vi "Reset Alarm.vi"(8 "error in (no error)":errorcluster, 11 "FujiMotor in":refnum<class "FujiMotor.lvclass">) -> (0 "error out":errorcluster, 3 "FujiMotor out":refnum<class "FujiMotor.lvclass">)   [LabVIEW 2014, in "ALPHA5 RS485.lvlib" / "FujiMotor.lvclass"]
uses:
  FujiMotor.lvclass
  FujiMotor.lvclass/FujiMotor.ctl
  ALPHA5 RS485.lvlib
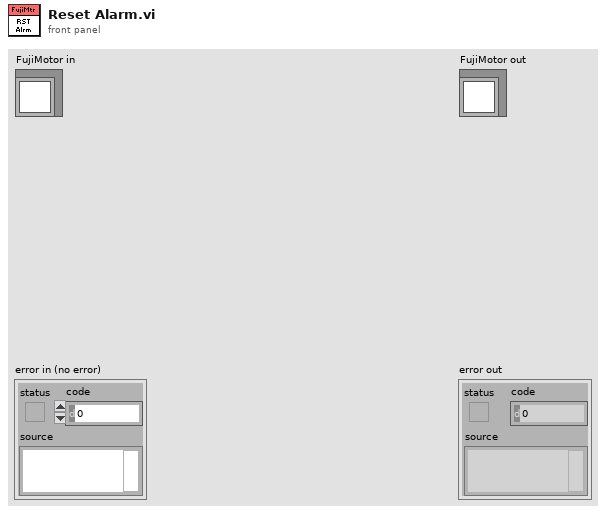
[diagram p1: front panel]
types:
  T1 = typedef "ALPHA5 RS485.lvlib/Port Selection Info.ctl" = cluster{"Port Name":refnum<visa-resource-name>, "Amplifier Num":u8, "Baud Rate":u32, "Char Formation":enum16{"0", "1", "2", "3", "4", "5"}}
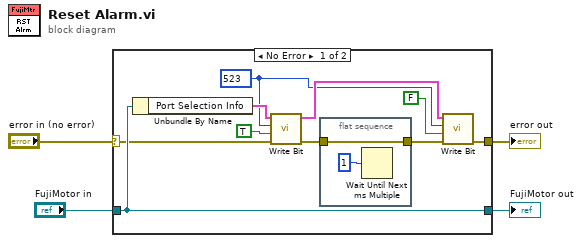
[diagram p0: block diagram]
diagram:
  n1 = case shown="No Error" "error in (no error)" {
    selector: "error in (no error)" -> [w12 w17]
    tunnel: [w7 w17] -> w3
    tunnel: [w14 w18] -> w1
    tunnel: "FujiMotor in" -> [w14 w18]
    frame No Error {
      w9 = u16 523 ("Address")
      n2 = Unbundle By Name(w14) -> ("Port Selection Info"=w13:T1)
      n3 = call "Write Bit.vi"("error in (no error)"=w12, "ON/OFF"=TRUE, "Address"=w9, "Port Selection Info In"=w13) -> ("error out"=w6:errorcluster, "Port Selection Info Out"=w10:T1)  [unwired: 6 in]
      n4 = flat-sequence {
        tunnel: w6 -> [w15]
        tunnel: [w15] -> w5
        frame #0 {
          n5 = Wait Until Next ms Multiple(millisecond multiple=u32 1) -> ()  [unwired: 1 out]
        }
      }
      n6 = call "Write Bit.vi"("error in (no error)"=w5, "ON/OFF"=FALSE, "Address"=w9, "Port Selection Info In"=w10) -> ("error out"=w7:errorcluster)  [unwired: 6 in, 1 out]
    }
    frame Error {
    }
  }
  "error out" <- w3
  "FujiMotor out" <- w1
